vi "Configure Multi Eval Meas List Segment Sequence Generation.vi"(0 "VISA resource name":refnum<visa-resource-name>, 1 "Allocation (1)":T1=1, 2 "DMRS ID (0)":i32, 5 "Instance (1)":T3=1, 7 "Segment (1)":i32=1, 9 "CC (1)":T2=1, 11 "error in (no error)":errorcluster, 12 "Initialization (Physical Cell ID Used)":i32(ring) items=["Physical Cell ID Used", "DMRS ID Used"], 13 "nSCID (0)":i32) -> (4 "VISA resource name out":refnum<visa-resource-name>, 15 "error out":errorcluster)   [LabVIEW 2020, in "Rohde&Schwarz CMWXP NR FR1 Measurement.lvlib"]
doc: "Configures the initialization of the DM-RS sequence generation, for carrier <cc>, allocation <a> in segment <no>.\n\nAttribute:\nRSCMWXPNRFR1M_ATTR_MULTI_EVAL_MEAS_LIST_SEGMENT_SEQUENCE_GENERATION\n\nRemote-control command:\nCONFigure:NRSub:MEAS<i>:LIST:SEGMent<no>[:CC<cc>]:ALLocation<a>:PUSCh:SGENeration"
uses:
  <instrlib>/Rohde&Schwarz CMWXP NR FR1 Measurement/Rohde&Schwarz CMWXP NR FR1 Measurement.lvlib
  <instrlib>/Rohde&Schwarz CMWXP NR FR1 Measurement/Private/_Instance.ctl
  <instrlib>/Rohde&Schwarz CMWXP NR FR1 Measurement/Private/_Carrier Component.ctl
  <instrlib>/Rohde&Schwarz CMWXP NR FR1 Measurement/Private/_Allocation.ctl
  <instrlib>/Rohde&Schwarz CMWXP NR FR1 Measurement/Private/rsidr_core.llb/rsidr_core.lvlib
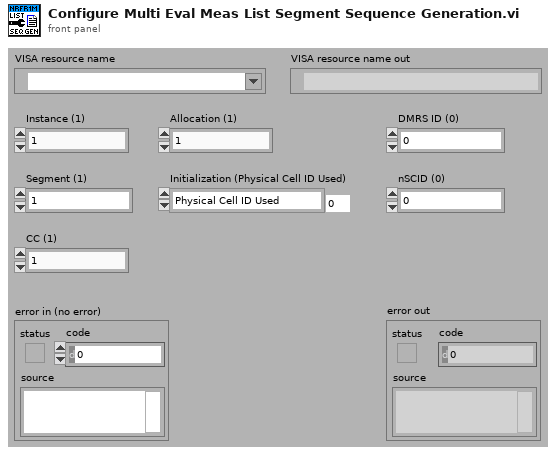
[diagram p1: front panel]
types:
  T1 = typedef "Rohde&Schwarz CMWXP NR FR1 Measurement.lvlib/_Allocation.ctl" = i32
  T2 = typedef "Rohde&Schwarz CMWXP NR FR1 Measurement.lvlib/_Carrier Component.ctl" = i32
  T3 = typedef "Rohde&Schwarz CMWXP NR FR1 Measurement.lvlib/_Instance.ctl" = i32
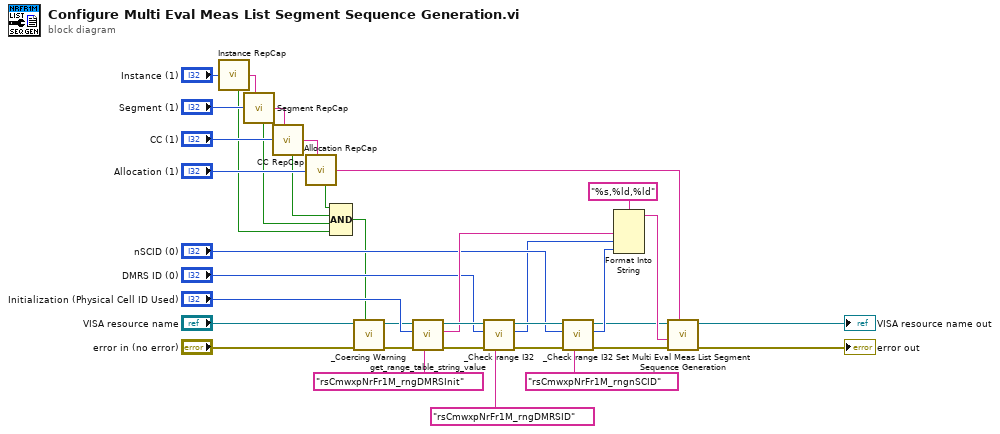
[diagram p0: block diagram]
diagram:
  n1 = call <instrlib>:"Instance RepCap.vi"("Instance In"="Instance (1)") -> ("In Range?"=w9:bool, "RepCap Identifier Out"=w32:string)  [unwired: 1 in]
  n2 = call <instrlib>:"Segment RepCap.vi"("Segment In"="Segment (1)", "RepCap String In (\"\")"=w32) -> ("In Range?"=w8:bool, "RepCap Identifier Out"=w31:string)
  n3 = call <instrlib>:"CC RepCap.vi"("CC In"="CC (1)", "RepCap String In (\"\")"=w31) -> ("In Range?"=w7:bool, "RepCap Identifier Out"=w29:string)
  n4 = call <instrlib>:"Allocation RepCap.vi"("Allocation In"="Allocation (1)", "RepCap String In (\"\")"=w29) -> ("In Range?"=w6:bool, "RepCap Identifier Out"=w27:string)
  n5 = Compound Arithmetic op=AND(w6, w7, w8, w9) -> (w1:bool)
  n6 = call <instrlib>:"_Coercing Warning.vi"("In Range?"=w1, "error in (no error)"="error in (no error)", "VISA resource name"="VISA resource name") -> ("error out"=w3:errorcluster, "VISA resource name out"=w2:refnum<visa-resource-name>)  [unwired: 7 in]
  n7 = call <instrlib>:"get_range_table_string_value.vi"("Range Table ID in"="rsCmwxpNrFr1M_rngDMRSInit", "error in"=w3, "I32 input"="Initialization (Physical Cell ID Used)", "VISA resource name"=w2) -> ("error out"=w25:errorcluster, "String Value out"=w20:string, "VISA resource name out"=w24:refnum<visa-resource-name>)  [unwired: 5 in]
  n8 = call <instrlib>:"_Check range I32.vi"("Range Table Identifier"="rsCmwxpNrFr1M_rngDMRSID", "error in (no error)"=w25, "I32 Value In"="DMRS ID (0)", "VISA resource name"=w24) -> ("error out"=w23:errorcluster, "I32 Value Out"=w17:i32, "VISA resource name out"=w22:refnum<visa-resource-name>)  [unwired: 5 in]
  n9 = call <instrlib>:"_Check range I32.vi"("Range Table Identifier"="rsCmwxpNrFr1M_rngnSCID", "error in (no error)"=w23, "I32 Value In"="nSCID (0)", "VISA resource name"=w22) -> ("error out"=w10:errorcluster, "I32 Value Out"=w16:i32, "VISA resource name out"=w11:refnum<visa-resource-name>)  [unwired: 5 in]
  n10 = Format Into String(format string="%s,%ld,%ld", w20, w17, w16) -> (resulting string=w12:string)  [unwired: 2 in, 1 out]
  n11 = call "Set Multi Eval Meas List Segment Sequence Generation"("Repeated Capabilities"=w27, "error in (no error)"=w10, "Multi Eval Meas List Segment Sequence Generation ()"=w12, "instrument handle"=w11) -> ("error out"=→"error out":errorcluster, "instrument handle out"=→"VISA resource name out":refnum<visa-resource-name>)  [unwired: 6 in]
